vi "Dashboard Main.vi"() -> ()   [LabVIEW 2014]
uses:
  <vilib>/event_ctls.llb/eventvkey.ctl
  <vilib>/Rock Robotics/WPI/Dashboard/WPI_DashboardLogging Global.vi
  <vilib>/Utility/config.llb/Write Key (String).vi
  <vilib>/Utility/config.llb/Write Key (I32).vi
  <vilib>/Utility/config.llb/NI_LVConfig.lvlib
panel:
  in  "TCP":refnum<k5>
  in  "Rec Mode":enum32{"Stop", "Record", "Playback"}(radio)
  in  "Vision":u16(ring) items=["Camera Off", "USB Camera SW", "USB Camera HW", "IP Camera"]
  out "Camera IP":string
  out "Image Message":string="Timeout in Camera Communications"
  in  "Dashboard Tab":T1(tab)
  in  "Camera Settings":T2={"Frame Rate"=30, "Compression"=30, "Size"=1} {"Frame Rate" scale=1.0..30.0; "Size" items=["640x480", "320x240", "160x120"]}
  out "MotorChart R":cluster{"Numeric":dbl, "Numeric":dbl}(graph)
  out "MotorChart L":T3(graph)
  out "MotorSliders R":cluster{"MotorSlide1":dbl, "MotorSlide2":dbl} {"MotorSlide2" scale=-1.0..1.0 scale format="%#_2e"; "MotorSlide1" scale=-1.0..1.0 scale format="%#_2e"}
  out "MotorSliders L":T4 {"MotorSlide4 2" scale=0.0..14.0 scale format="%#_2e"; "MotorSlide2" scale=-1.0..1.0 scale format="%#_2e"; "MotorSlide1" scale=-1.0..1.0 scale format="%#_2e"}
  out "JS1 Z":dbl(slide) scale=-1.0..1.0 scale format="%#_2e"
  out "JS1 Graph":cluster{"X":dbl, "Y":dbl}[](graph)
  out "JS1 Buttons":T5
  out "JS2 Z":dbl(slide) scale=-1.0..1.0 scale format="%#_2e"
  out "JS2 Graph":cluster{"X":dbl, "Y":dbl}[](graph)
  out "JS2 Buttons":T5
  out "Mode":T6(ring)=enum."Auto Disabled"
  in  "DB Camera Config":bool
  out "fps":dbl format="%#.1g"
  out "Mbps":dbl format="%#.1g"
  out "Mbps 2":bool
  in  "DB/String 9":string
  in  "DB/String 8":string
  in  "DB/String 7":string
  in  "DB/String 6":string
  in  "DB/String 5":string
  in  "DB/String 4":string
  in  "DB/String 3":string
  in  "DB/String 2":string
  in  "DB/String 1":string
  in  "DB/String 0":string
  in  "DB/Slider 0":dbl(slide) scale=0.0..5.0
  in  "DB/Slider 1":dbl(slide) scale=0.0..5.0
  in  "DB/Slider 2":dbl(slide) scale=0.0..5.0
  in  "DB/Slider 3":dbl(slide) scale=0.0..5.0
  out "DB/LED 3":bool
  out "DB/LED 2":bool
  out "DB/LED 1":bool
  out "DB/LED 0":bool
  in  "DB/Button 3":bool
  in  "DB/Button 2":bool
  in  "DB/Button 1":bool
  in  "DB/Button 0":bool caption="New Name"
  in  "Test Slider":dbl(slide) scale=0.0..100.0 scale format="%#_3g"
  in  "On/Off":bool caption="Solenoid"
  in  "Test Name":u16(ring) items=["Select the test to run...", "Example Test", "-------------------------------", "List of tests is built in robot code.", "Replace with your own automated tests."]
  in  "Test Tree":string(tree)
  in  "Motor":cluster{"Value":dbl, "Enable":bool} {"Value" scale=-1.0..1.0 scale format="%#_3g"}
  out "Progress":T7 {"Test Progress" scale=0.0..100.0}
  in  "Rev/Fwd":cluster{"Forward":bool, "Reverse":bool}
  in  "Test Ring":u16(ring) items=["Monochrome", "Color"]
  in  "Listbox":i32(listbox)
  out "Tree":string(tree)
  out "Camera Image":T8(plugin-control)
  out "Boolean":bool
  # "Left"
  # "Front"
  # "Right"
  # "Battery"
  # "v 1.0"
  # "This tab is a great place for autonomous settings and robot-specific values.\nPlace controls and indicators inside this tab and match name to\nDashboard Variables on robot. You can also delete this comment."
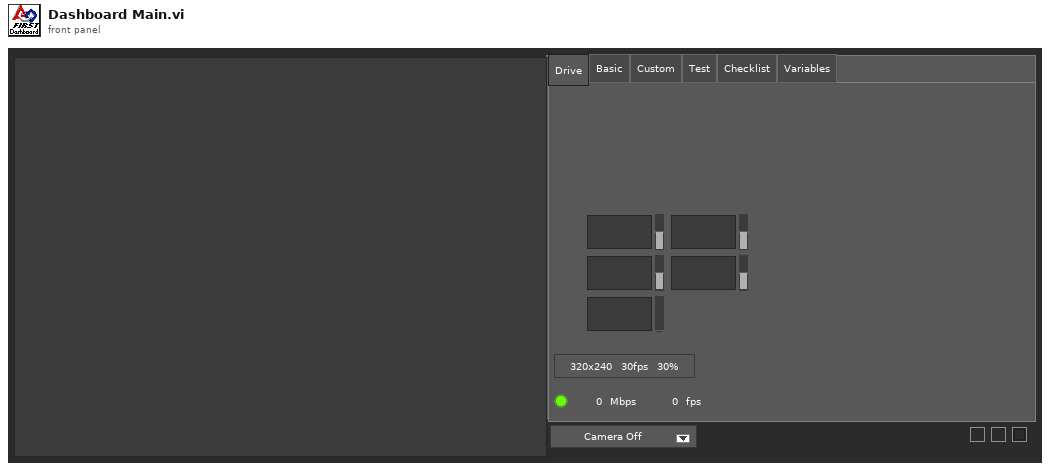
[diagram p1: front panel]
types:
  T1 = enum32{"Drive", "Basic", "Custom", "Test", "Checklist", "Variables"}
  T2 = cluster{"Frame Rate":i32, "Compression":i32, "Size":u16}
  T3 = cluster{"Numeric":dbl, "Numeric":dbl, "Battery V":dbl}
  T4 = cluster{"MotorSlide1":dbl, "MotorSlide2":dbl, "MotorSlide4 2":dbl}
  T5 = cluster{bool, bool, bool, bool, bool, bool, bool, bool, bool, bool, bool, bool}
  T6 = enum8{"Tele-Op Disabled", "Tele-Op Enabled", "Auto Disabled", "Auto Enabled", "Test Disabled", "Test Enabled", "Disconnected", "No Code", "E-Stop"}
  T7 = cluster{"Test Progress":u8, "Test Progress Text":string}
  T8 = typedef "IMAQ Image.ctl" = refnum<image>
  T9 = typedef "Image Type" = u32
  T10 = cluster{"Camera Image":refnum<vi>, "Dashboard Tab":refnum<vi>, "Boolean":refnum<vi>, "Vision":refnum<vi>, "Rec Mode":refnum<vi>, "Test Slider":refnum<vi>, "On/Off ":refnum<vi>, "Test Ring":refnum<vi>, "Rev/Fwd":refnum<vi>, "Test Name":refnum<vi>, "Motor":refnum<vi>, "Progress":refnum<vi>, "CheckList":refnum<vi>, "Tree":refnum<vi>, "Test Tree":refnum<vi>}
  T11 = cluster{"Error Strings":string, "Disable Counts":cluster{u16, u16}, "Rail Faults":cluster{u16, u16, u16}, "Robot IP":string, "DB Mode":u8, "Event Info":cluster{"Name":string, "Type":u8, "Number":u16, "Replay":u8}, "Camera Addr":string}
  T12 = cluster{"Storage":cluster{"Disk Free":u64, "RAM Block":u32, "RAM free":u32}, "CPU Utilization":cluster{"CPU % ISR":sgl, "CPU % Time Crit":sgl, "CPU % Timed Str":sgl, "CPU % High":sgl, "CPU % Above":sgl, "CPU % Normal":sgl, "CPU % Low":sgl}, "CAN":cluster{"% Bus Utilization":sgl, "Bus Off Cnt":u32, "TX_FIFO Full Cnt":u32, "Receive Error Cnt":u8, "Transmit Error Cnt":u8}, "HID":cluster{"HID Outputs":u32, "Rumble Low":u16, "Rumble High":u16}[]}
  T13 = cluster{"Status bits":cluster{"Test Mode":bool, "Autonomous":bool, "Enabled":bool, "Code Start":bool, "Brownout":bool, "Reserved 2":bool, "Reserved 3":bool, "E-Stop":bool}, "Code Trace":cluster{"Disabled":bool, "TeleOp":bool, "Auto":bool, "Test":bool}, "Controller Type":enum16{"unknown", "cRIO", "roboRio"}, "Code?":enum16{"unknown", "noCode", "code"}, "Battery V":dbl}
  T14 = cluster{"Control Bits":cluster{"TestMode":bool, "Autonomous":bool, "Enabled":bool, "FMS Present":bool, bool, bool, bool, "E-Stop":bool}, "Team Station ":u8, "Countdown":sgl, "Joystick Values":cluster{"Axes":dbl[], "Buttons":bool[], "POVs":i16[]}[]}
  T15 = cluster{"Axes":dbl[], "Buttons":bool[], "POVs":i16[]}[]
  T16 = cluster{"Axes":dbl[], "Buttons":bool[], "POVs":i16[]}
  T17 = cluster{"Buttons[0]":bool, "Buttons[1]":bool, "Buttons[2]":bool, "Buttons[3]":bool, "Buttons[4]":bool, "Buttons[5]":bool, "Buttons[6]":bool, "Buttons[7]":bool, "Buttons[8]":bool, "Buttons[9]":bool, "Buttons[10]":bool, "Buttons[11]":bool}
  T18 = typedef "NI_LVConfig.lvlib/Config Data RefNum.ctl" = refnum<k1>
  T19 = cluster{"Operation":enum16{"Update", "Clear"}, "Color Box":u32}[]
  T20 = typedef "eventvkey.ctl" = enum16{"ASCII", "Enter", "Return", "Shift", "Ctrl", "Alt", "Cmd", "Opt", "Caps", "NumLock", "Clear", "Break", "Up", "Down", "Left", "Right", "Insert", "Delete", "Home", "End", "PageUp", "PageDown", "Escape", "Help", "Pause", "ScrollLock", "F1", "F2", "F3", "F4", "F5", "F6", "F7", "F8", "F9", "F10", "F11", "F12", "F13", "F14", "F15", "F16", "F17", "F18", "F19", "F20", "F21", "F22", "F23", "F24", "Play", "VolumeUp", "VolumeDown", "Mute", "Two Byte Char"}
  T21 = cluster{"Image Size":bool, "Image Type":bool, "Pixel Value":bool, "ROI Information":bool, "Zoom Factor":bool}
  T22 = enum8{"Enabled", "Disabled", "Disabled and Grayed Out"}
  T23 = cluster{"Operation":enum16{"Update", "Clear"}, "Color Box":u32}
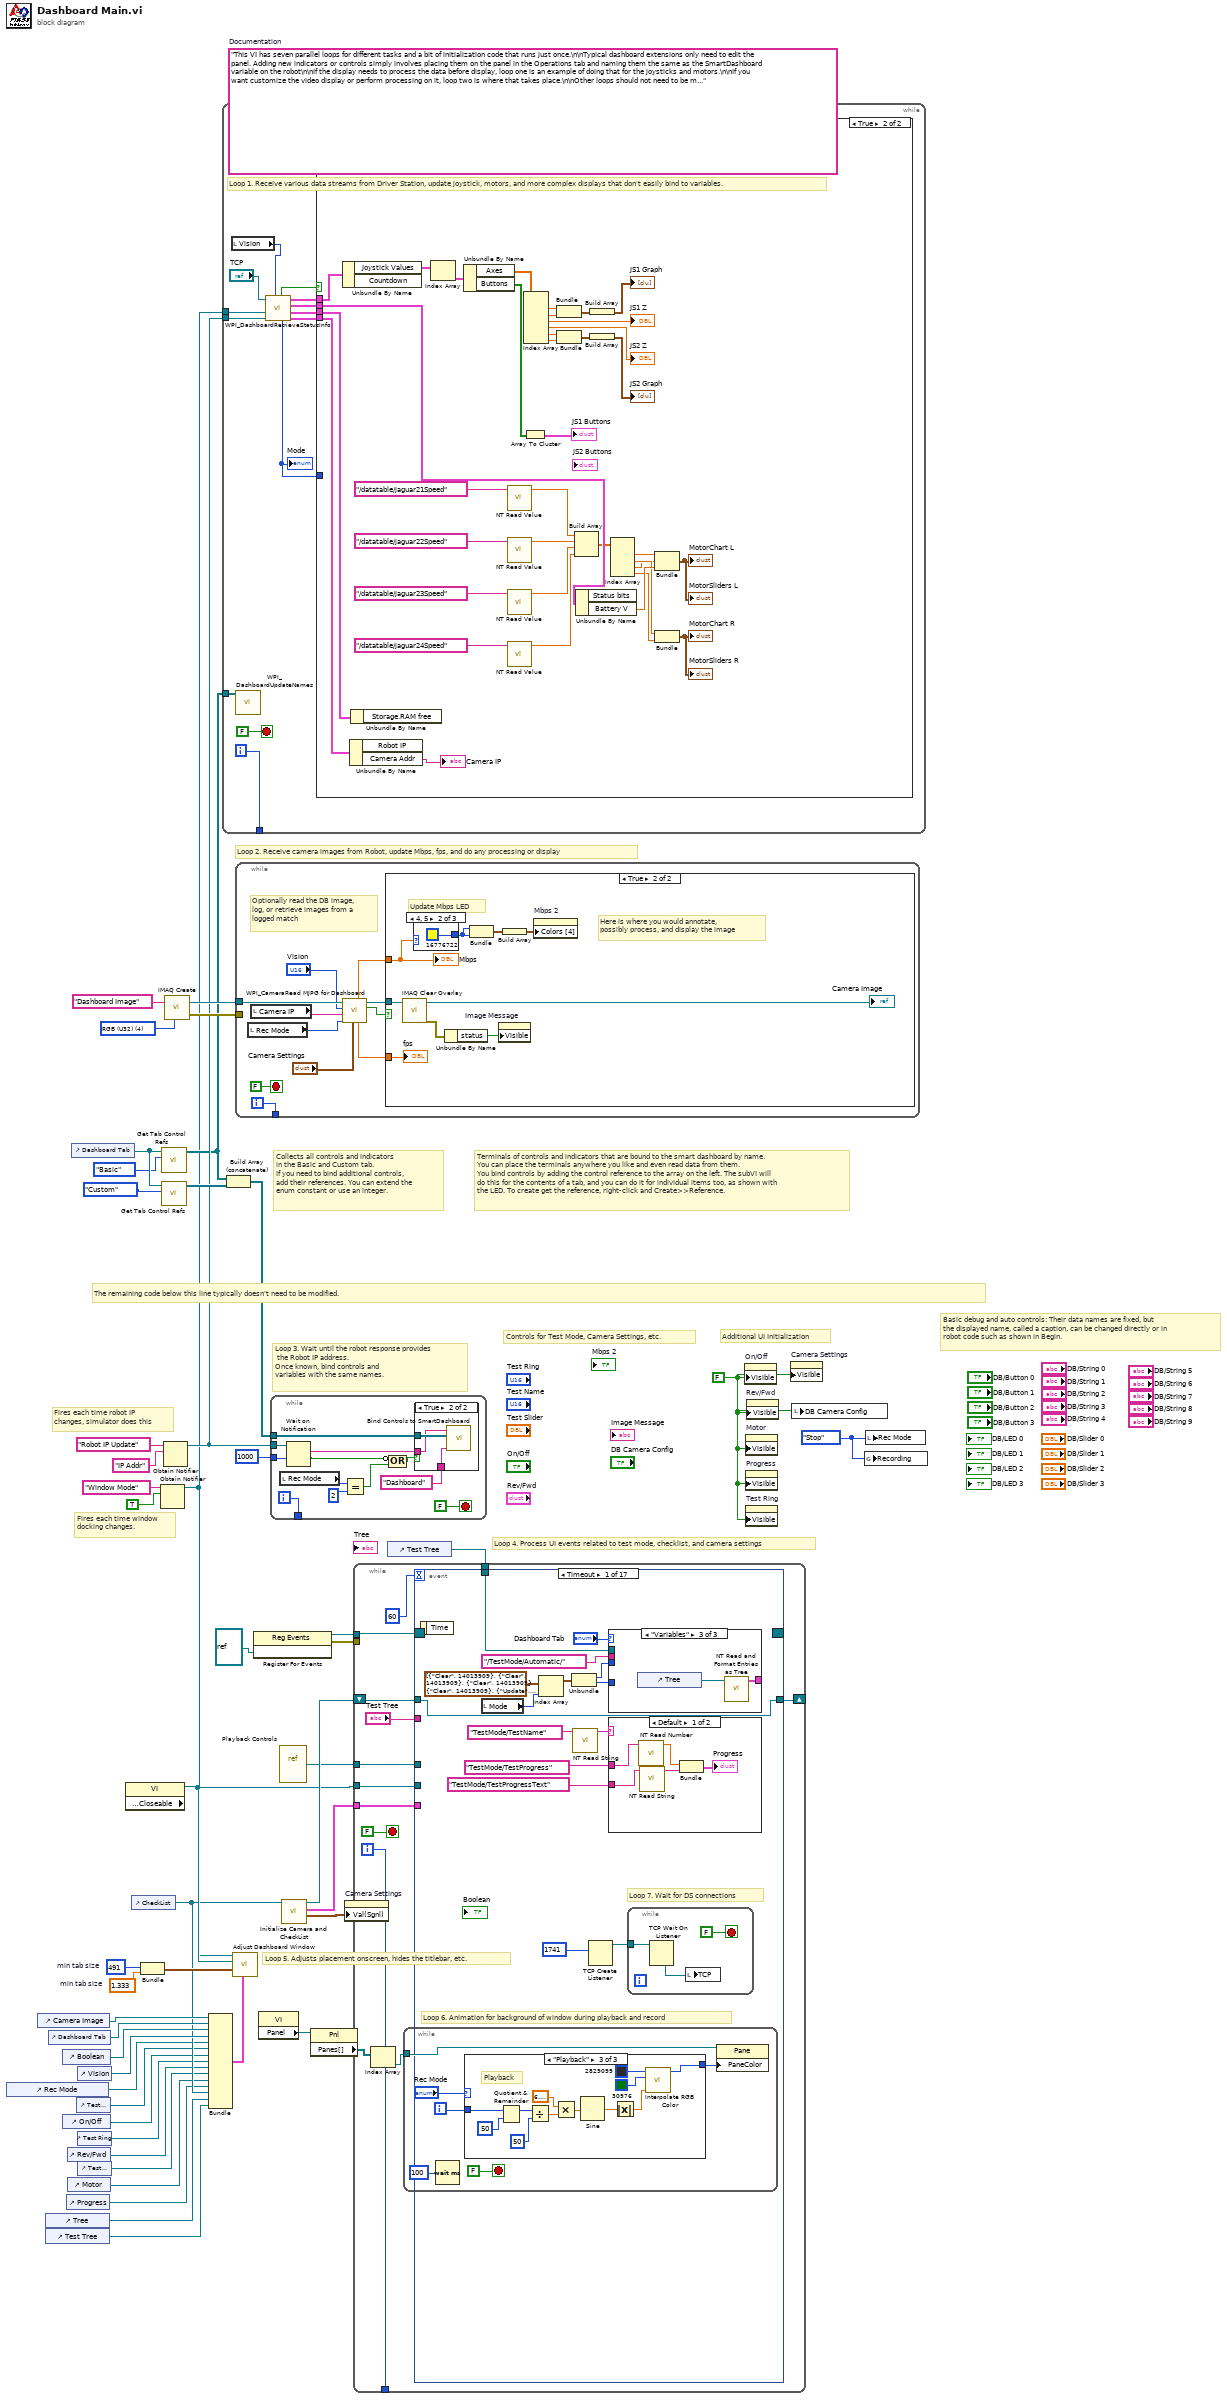
[diagram p0: block diagram]
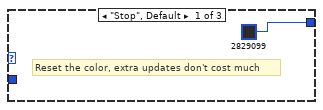
[diagram p3: hidden frame]
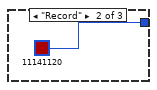
[diagram p4: hidden frame]
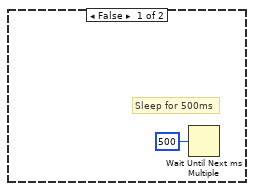
[diagram p6: hidden frame]
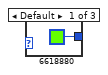
[diagram p7: hidden frame]
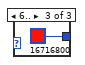
[diagram p8: hidden frame]
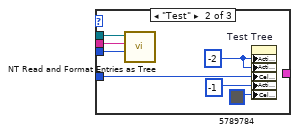
[diagram p10: hidden frame]
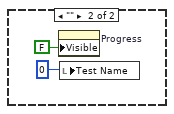
[diagram p11: hidden frame]
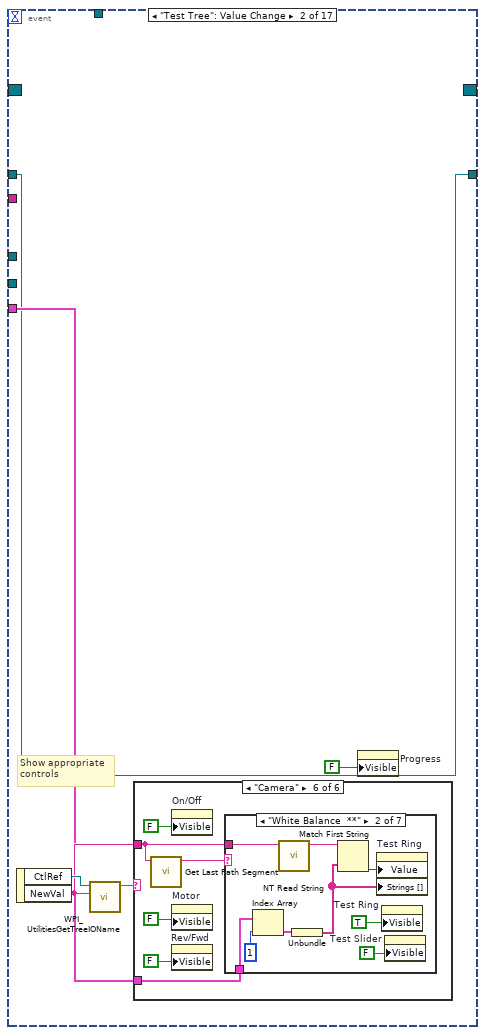
[diagram p12: hidden frame]
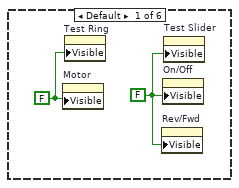
[diagram p13: hidden frame]
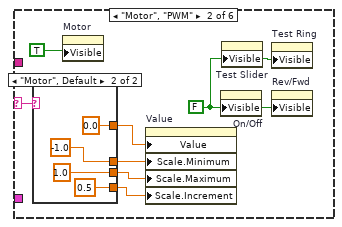
[diagram p14: hidden frame]
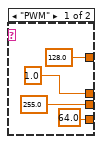
[diagram p15: hidden frame]
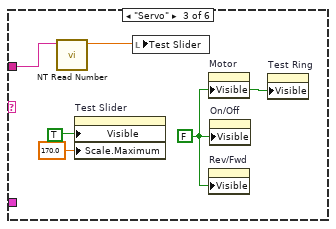
[diagram p16: hidden frame]
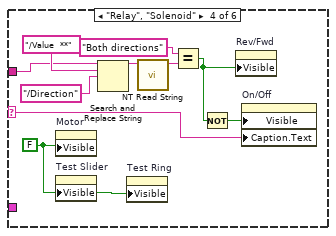
[diagram p17: hidden frame]
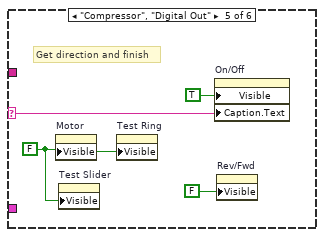
[diagram p18: hidden frame]
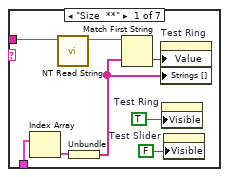
[diagram p19: hidden frame]
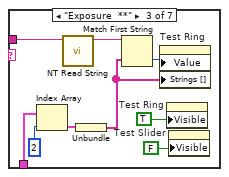
[diagram p20: hidden frame]
diagram:
  w24 = 491  # min tab size
  w23 = 1.333  # min tab size
  w32 = enum32{"Stop", "Record", "Playback"}."Stop" ("Rec Mode")
  w6 = FALSE ("Visible")
  (unwired) "This VI has seven parallel loops for different tasks and a bit of initialization code that runs just once.\n\nTypical dashboard extensions only need to edit the panel. Adding new indicators or controls simply involves placing them on the panel in the Operations tab and naming them the same as the SmartDashboard variable on the robot\n\nIf the display needs to process the data before display, loop one is an example of doing that for the joysticks and motors.\n\nIf you want customize the video display or perform processing on it, loop two is where that takes place.\n\nOther loops should not need to be modified. They are pretty standard, and document the task they perform."  # Documentation
  w52 = T9 4 items=["Grayscale (U8)", "Grayscale (I16)", "Grayscale (SGL)", "Complex (CSG)", "RGB (U32)", "HSL (U32)", "RGB (U64)"] ("Image Type")
  # "Loop 7. Wait for DS connections"
  # "Basic debug and auto controls: Their data names are fixed, but\nthe displayed name, called a caption, can be changed directly or in\nrobot code such as shown in Begin."
  # "Controls for Test Mode, Camera Settings, etc."
  # "Additional UI Initialization"
  # "Loop 6. Animation for background of window during playback and record"
  # "Fires each time robot IP\nchanges, simulator does this"
  # "Fires each time window\ndocking changes."
  # "Collects all controls and indicators\nin the Basic and Custom tab.\nIf you need to bind additional controls,\nadd their references. You can extend the\nenum constant or use an integer."
  # "The remaining code below this line typically doesn't need to be modified."
  # "Loop 4. Process UI events related to test mode, checklist, and camera settings"
  # "Terminals of controls and indicators that are bound to the smart dashboard by name.\nYou can place the terminals anywhere you like and even read data from them.\nYou bind controls by adding the control reference to the array on the left. The subVI will\ndo this for the contents of a tab, and you can do it for individual items too, as shown with\nthe LED. To create get the reference, right-click and Create>>Reference."
  # "Loop 3. Wait until the robot response provides\n the Robot IP address.\nOnce known, bind controls and\nvariables with the same names."
  # "Loop 5. Adjusts placement onscreen, hides the titlebar, etc."
  # "Loop 1. Receive various data streams from Driver Station, update joystick, motors, and more complex displays that don't easily bind to variables."
  # "Loop 2. Receive camera images from Robot, update Mbps, fps, and do any processing or display"
  n1 = control-ref of="Rec Mode"() -> (w12:refnum<vi>)
  n2 = control-ref of="Camera Image"() -> (w27:refnum<vi>)
  n3 = control-ref of="Tree"() -> (w16:refnum<vi>)
  n4 = control-ref of="Test Tree"() -> (w15:refnum<vi>)
  n5 = control-ref of="Dashboard Tab"() -> (w26:refnum<vi>)
  n6 = control-ref of="Boolean"() -> (w21:refnum<vi>)
  n7 = control-ref of="On/Off"() -> (w10:refnum<vi>)
  n8 = control-ref of="Progress"() -> (w7:refnum<vi>)
  n9 = control-ref of="Rev/Fwd"() -> (w8:refnum<vi>)
  n10 = control-ref of="Motor"() -> (w13:refnum<vi>)
  n11 = control-ref of="Dashboard Tab"() -> (w30:refnum<vi>)
  n12 = control-ref of="Test Slider"() -> (w11:refnum<vi>)
  n13 = control-ref of="Vision"() -> (w25:refnum<vi>)
  n14 = control-ref of="Test Ring"() -> (w9:refnum<vi>)
  n15 = control-ref of="Test Name"() -> (w14:refnum<vi>)
  n16 = property class="VI" props=["Front Panel.Closeable"]() -> (reference out=w31:refnum<vi>)  [unwired: 2 in, 2 out]
  n17 = control-ref of="CheckList"() -> (w17:refnum<vi>)
  n18 = Bundle("min tab size"=w24, "min tab size"=w23) -> (w22:cluster{"min tab size":i32, "min tab size":dbl})  [unwired: 1 in]
  n19 = Obtain Notifier(name (unnamed)="Window Mode", notification data type=TRUE) -> (notifier out=w3:refnum<notifier>)  [unwired: 2 in, 2 out]
  n20 = call <vilib>:"Get Tab Control Refs.vi"("Page Index"=T1."Basic" ("Dashboard Tab"), "TabControl in"=w30) -> ("ControlsOnPage"=w4:refnum<vi>[])  [unwired: 9 in]
  n21 = call <vilib>:"Get Tab Control Refs.vi"("Page Index"=T1."Custom" ("Dashboard Tab"), "TabControl in"=w30) -> ("ControlsOnPage"=w29:refnum<vi>[])  [unwired: 9 in]
  n22 = Obtain Notifier(name (unnamed)="Robot IP Update", notification data type="IP Addr" ("name (unnamed)")) -> (notifier out=w5:refnum<notifier>)  [unwired: 2 in, 2 out]
  n23 = call "IMAQ Create"("Image Name"="Dashboard Image", "Image Type"=w52) -> ("New Image"=w50:T8, "error out"=w49:errorcluster)  [unwired: 2 in, 1 out]
  n24 = Bundle("Camera Image"=w27, "Dashboard Tab"=w26, "Boolean"=w21, "Vision"=w25, "Rec Mode"=w12, "Test Slider"=w11, "On/Off"=w10, "Test Ring"=w9, "Rev/Fwd"=w8, "Test Name"=w14, "Motor"=w13, "Progress"=w7, "CheckList"=w17, "Tree"=w16, "Test Tree"=w15) -> (w18:T10)  [unwired: 1 in]
  n25 = while {
    tunnel: [w64] -> _
    tunnel: w5 -> [w58]
    tunnel: w4 -> [w57]
    tunnel: w3 -> [w53]
    i -> [w64]
    stop <- FALSE stop-if-true
    n26 = local read "Vision"() -> (w55:u16)
    n27 = call <vilib>:"WPI_DashboardUpdateNames.vi"("Controls on Tab"=w57) -> ()  [unwired: 11 in]
    n28 = call <vilib>:"WPI_DashboardRetrieveStatusInfo.vi"("Vision"=w55, "Binding Refnum"=w58, "Window Mode Notifier"=w53, "TCP Cnx"="TCP") -> ("Power and Errors"=w59:T11, "Robot Metrics"=w62:T12, "Status Info"=w63:T13, "Control Info"=w60:T14, "Robot Mode"=w56:T6, "Process?"=w61:bool)  [unwired: 2 in]
    "Mode" <- w56
    n29 = case shown="True" w61 {
      tunnel: w63 -> [_ w101]
      tunnel: w62 -> [_ w100]
      tunnel: w60 -> [_ w99]
      tunnel: w59 -> [_ w98]
      tunnel: w56 -> [_ _]
      frame False {
      }
      frame True {
        n30 = Unbundle By Name(w99) -> ("Joystick Values"=w94:T15)  [unwired: 1 out]
        n31 = Unbundle By Name(w98) -> ("Camera Addr"=→"Camera IP":string)  [unwired: 1 out]
        n32 = Unbundle By Name(w100) -> ()  [unwired: 1 out]
        n33 = Index Array(array=w94) -> (element=w92:T16)  [unwired: 1 in]
        n34 = Unbundle By Name(w92) -> ("Axes"=w88:dbl[], "Buttons"=w87:bool[])
        n35 = call-poly <vilib>:"NT Read Value.vi"("Name"="/datatable/jaguar21Speed") -> ("Numeric"=w74:dbl)  [unwired: 9 in, 1 out]
        n36 = call-poly <vilib>:"NT Read Value.vi"("Name"="/datatable/jaguar22Speed") -> ("Numeric"=w73:dbl)  [unwired: 9 in, 1 out]
        n37 = call-poly <vilib>:"NT Read Value.vi"("Name"="/datatable/jaguar23Speed") -> ("Numeric"=w71:dbl)  [unwired: 9 in, 1 out]
        n38 = call-poly <vilib>:"NT Read Value.vi"("Name"="/datatable/jaguar24Speed") -> ("Numeric"=w70:dbl)  [unwired: 9 in, 1 out]
        n39 = Array To Cluster(array=w87) -> (cluster=→"JS1 Buttons":T17)
        n40 = Index Array(array=w88) -> (element #1=w90:dbl, element #2=w91:dbl, element #3=→"JS1 Z":dbl, element #4=→"JS2 Z":dbl, element #5=w67:dbl, element #6=w66:dbl)  [unwired: 6 in]
        n41 = Bundle("X axis"=w90, "X axis"=w91) -> (w89:cluster{"X axis":dbl, "X axis":dbl})  [unwired: 1 in]
        n42 = Bundle("X axis"=w67, "X axis"=w66) -> (w84:cluster{"X axis":dbl, "X axis":dbl})  [unwired: 1 in]
        n43 = Build Array(w74, w73, w71, w70) -> (w72:dbl[])
        n44 = Unbundle By Name(w101) -> ("Battery V"=w95:dbl)  [unwired: 1 out]
        n45 = Build Array(w89) -> (→"JS1 Graph":cluster{"X axis":dbl, "X axis":dbl}[])
        n46 = Build Array(w84) -> (→"JS2 Graph":cluster{"X axis":dbl, "X axis":dbl}[])
        n47 = Index Array(array=w72) -> (element #1=w82:dbl, element #2=w81:dbl, element #3=w80:dbl, element #4=w79:dbl)  [unwired: 4 in]
        n48 = Bundle("Numeric"=w82, "Numeric"=w80, "Battery V"=w95) -> (→"MotorChart L" →"MotorSliders L":T3)  [unwired: 1 in]
        n49 = Bundle("Numeric"=w81, "Numeric"=w79) -> (→"MotorChart R" →"MotorSliders R":cluster{"Numeric":dbl, "Numeric":dbl})  [unwired: 1 in]
      }
    }
  }
  n50 = Build Array (concatenate)(w4, w29) -> (w28:refnum<vi>[])
  n51 = call "Adjust Dashboard Window.vi"("Sizing Refnums"=w18, "Size Constraints"=w22, "VI"=w31, "Notifier in"=w3) -> ()  [unwired: 8 in]
  n52 = while {
    tunnel: w50 -> [w110]
    tunnel: w49 -> [_]
    tunnel: [w111] -> _
    i -> [w111]
    stop <- FALSE stop-if-true
    # "Optionally read the DB image,\nlog, or retrieve images from a\nlogged match"
    n53 = local read "Rec Mode"() -> (w104:enum32{"Stop", "Record", "Playback"})
    n54 = local read "Camera IP"() -> (w102:string)
    n55 = call <vilib>:"WPI_CameraRead MJPG for Dashboard.vi"("Camera Settings"="Camera Settings", "Rec Mode"=w104, "Camera IP"=w102, "Camera Mode"="Vision", "Refnum in"=w110) -> ("Active"=w108:bool, "Refnum out"=w109:T8, "FPS"=w107:dbl, "Bandwidth (Mbps)"=w106:dbl)  [unwired: 3 in]
    n56 = case shown="True" w108 {
      tunnel: w109 -> [_ w117]
      tunnel: w106 -> [_ w116]
      tunnel: w107 -> [_ w114]
      frame False {
        # "Sleep for 500ms"
        n57 = Wait Until Next ms Multiple(millisecond multiple=u32 500) -> ()  [unwired: 1 out]
      }
      frame True {
        # "Here is where you would annotate,\npossibly process, and display the image"
        # "Update Mbps LED"
        n58 = call "IMAQ Clear Overlay"("Image"=w117) -> ("error out"=w121:errorcluster, "Image Out"=→"Camera Image":T8)  [unwired: 2 in, 7 out]
        n59 = case shown="4, 5" w116 {
          tunnel: [u32 6618880 ("Color Box") u32 16776722 ("Color Box") u32 16716800 ("Color Box")] -> w118
          frame Default {
          }
          frame 4, 5 {
          }
          frame 6.. {
          }
        }
        n60 = Unbundle By Name(w121) -> ("status"=w122:bool)
        n61 = Bundle("Color Box"=w118, "Color Box"=w118) -> (w120:cluster{"Color Box":u32, "Color Box":u32})  [unwired: 1 out]
        n62 = property on="Image Message" class="Str"("Visible"=w122) -> ()  [unwired: 2 in, 2 out]
        n63 = Build Array(w120) -> (w119:cluster{"Color Box":u32, "Color Box":u32}[])
        n64 = property on="Mbps 2" class="Bool (strict)"("Colors [4]"=w119) -> ()  [unwired: 2 in, 2 out]
        "Mbps" <- w116
        "fps" <- w114
      }
    }
  }
  n65 = register-events(refnum<vi> refnum) -> (reference out=w36:refnum<event-registration>, error out=w35:errorcluster)  [unwired: 2 in]
  n66 = property class="VI"() -> ("Panel"=w39:refnum<vi>)  [unwired: 2 in, 2 out]
  n67 = while {
    tunnel: w28 -> [w137]
    tunnel: w5 -> [w135]
    tunnel: [w133] -> _
    tunnel: u32 1000 ("milliseconds to wait") -> [w132]
    i -> [w133]
    stop <- FALSE stop-if-true
    n68 = local read "Rec Mode"() -> (w128:enum32{"Stop", "Record", "Playback"})
    n69 = Wait on Notification(notifier=w135, timeout in ms (-1)=w132) -> (notification=w134:string, timed out?=w130:bool)  [unwired: 2 in, 2 out]
    n70 = Equal?(x=w128, y=u16 2 ("Rec Mode")) -> (x = y?=w129:bool)
    n71 = Compound Arithmetic op=OR(invert w130, w129) -> (w131:bool)
    n72 = case shown="True" w131 {
      tunnel: w137 -> [_ w140]
      tunnel: w134 -> [_ w139]
      tunnel: "Dashboard" -> [_ w138]
      frame False {
      }
      frame True {
        n73 = call <vilib>:"Bind Controls to SmartDashboard.vi"("Client Name"=w138, "Bound Control Refs"=w140, "Server IP Address"=w139) -> ()  [unwired: 9 in]
      }
    }
  }
  n74 = vi-ref "Playback Controls.vi"() -> (w37:refnum<vi>)
  n75 = call "Initialize Camera and CheckList.vi"("ListBox in"=w17) -> ("Cluster"=w43:cluster{"value":i32, "value":i32, "index":i32}, "Array"=w44:cluster{string[]}[], "File Refnum"=w42:T18)  [unwired: 8 in]
  n76 = property class="Pnl"(reference=w39) -> ("Panes[]"=w40:refnum<vi>[])  [unwired: 1 in, 2 out]
  n77 = property on="Camera Settings" class="Clust (strict)"("Val(Sgnl)"=w43) -> ()  [unwired: 2 in, 2 out]
  n78 = Index Array(array=w40) -> (element=w38:refnum<vi>)  [unwired: 1 in]
  n79 = control-ref of="Test Tree"() -> (w41:refnum<vi>)
  n80 = while {
    tunnel: w44 -> [w148]
    shift-right: [w147] -> _
    shift-left: w42 -> [w146]
    tunnel: [w145] -> _
    tunnel: w41 -> [w144]
    tunnel: w37 -> [w143]
    tunnel: w36 -> [w142]
    tunnel: w35 -> [_]
    tunnel: w31 -> [w141]
    i -> [w145]
    stop <- FALSE stop-if-true
    n81 = event shown="[0] Timeout" {
      selector: w142 -> [_ _ _ _ _ _ _ _ _ _ _ _ _ _ _ _ _]
      dyn-events: [_ _ _ _ _ _ _ _ _ _ _ _ _ w386 _ _ _] -> _
      timeout: u32 60 ("milliseconds to wait") -> [_ _ _ _ _ _ _ _ _ _ _ _ _ _ _ _ _]
      tunnel: w144 -> [w160 _ _ _ _ _ _ _ _ _ _ _ _ _ _ _ _]
      tunnel: "Test Tree" -> [_ _ _ _ _ _ _ _ w355 w363 w365 w369 w377 _ _ _ _]
      tunnel: w148 -> [_ w182 _ _ _ _ w319 w349 _ _ _ _ _ _ _ _ _]
      tunnel: [w156 w181 w280 w285 w293 w305 w318 w342 w354 w361 w364 w368 w376 w388 w402 w403 w413] -> w147
      tunnel: w146 -> [w156 w181 w280 w285 w293 w305 w317 w342 w354 w361 w364 w368 w376 w388 w402 w403 w413]
      tunnel: w143 -> [_ _ _ _ _ _ _ _ _ _ _ _ _ w389 _ w406 _]
      tunnel: w141 -> [_ _ _ _ _ _ _ _ _ _ _ _ _ w384 _ _ _]
      event Timeout {
        n82 = event-data() -> ()  [unwired: 1 in, 1 out]
        n83 = local read "Mode"() -> (w159:T6)
        n84 = Index Array(array=T19 [{"Operation"=enum."Clear", "Color Box"=14013909}, {"Operation"=enum."Clear", "Color Box"=14013909}, {"Operation"=enum."Clear", "Color Box"=14013909}, {"Operation"=enum."Clear", "Color Box"=14013909}, {"Operation"=enum."Update", "Color Box"=14013909}, {"Operation"=enum."Update", "Color Box"=16777215}, {"Operation"=enum."Clear", "Color Box"=14013909}, {"Operation"=enum."Clear", "Color Box"=14013909}, {"Operation"=enum."Clear", "Color Box"=14013909}], index=w159) -> (element=w154:T23)
        n85 = Unbundle(w154) -> ("Operation"=w153:enum16{"Update", "Clear"}, "Color Box"=w152:u32)
        n86 = call <vilib>:"NT Read String.vi"("Name"="TestMode/TestName") -> ("String"=w163:string)  [unwired: 9 in, 1 out]
        n87 = case shown="\"Variables\"" "Dashboard Tab" {
          tunnel: w160 -> [_ w171 _]
          tunnel: "/TestMode/Automatic/" ("Name Pattern") -> [_ w170 _]
          tunnel: w153 -> [_ w169 _]
          tunnel: [_ _ w173] -> _
          tunnel: w152 -> [_ w165 _]
          frame "Custom", Default {
          }
          frame "Test" {
            w168 = -2 ("Active Item:Row Number")
            n88 = call <vilib>:"NT Read and Format Entries as Tree.vi"("Operation"=w169, "Name Pattern"=w170, "Tree Refnum"=w171) -> ()  [unwired: 7 in, 2 out]
            n89 = property on="Test Tree" class="Tree (strict)"("Active Item Row Number"=w168, "ActiveColNum"=w168, "CellBG"=w165, "Active Item Row Number"=-1 ("Active Item:Row Number"), "CellBG"=u32 5789784 ("Color Box")) -> ()  [unwired: 2 in, 2 out]
          }
          frame "Variables" {
            n90 = control-ref of="Tree"() -> (w172:refnum<vi>)
            n91 = call <vilib>:"NT Read and Format Entries as Tree.vi"("Tree Refnum"=w172) -> ("Formatted Strings"=w173:cluster{"Name":string, "Value":string}[])  [unwired: 9 in, 1 out]
          }
        }
        n92 = case shown="Default" w163 {
          tunnel: "TestMode/TestProgress" ("Name") -> [w175 _]
          tunnel: "TestMode/TestProgressText" ("Name") -> [w174 _]
          frame Default {
            n93 = call <vilib>:"NT Read Number.vi"("Name"=w175) -> ("Numeric"=w176:dbl)  [unwired: 9 in, 1 out]
            n94 = call <vilib>:"NT Read String.vi"("Name"=w174) -> ("String"=w177:string)  [unwired: 9 in, 1 out]
            n95 = Bundle("Numeric"=w176, "String"=w177) -> (→"Progress":cluster{"Numeric":dbl, "String":string})  [unwired: 1 in]
          }
          frame "" {
            n96 = property on="Progress" class="Clust (strict)"("Visible"=FALSE) -> ()  [unwired: 2 in, 2 out]
            n97 = local write "Test Name"(u16 0) -> ()
          }
        }
      }
      event "Test Tree": Value Change {
        # "Show appropriate\ncontrols"
        n98 = event-data() -> ("CtlRef"=w185:refnum<vi>, "NewVal"=w183:string)  [unwired: 1 in]
        n99 = call <vilib>:"WPI_UtilitiesGetTreeIOName.vi"("NewVal"=w183, "TreeControl in"=w185) -> ("I/O Name"=w186:string)  [unwired: 9 in]
        n100 = case shown="\"Camera\"" w186 {
          selector: w186 -> [_ w193 _ w211 w220 _]
          tunnel: w183 -> [_ _ w208 w210 _ w227]
          tunnel: w182 -> [_ _ _ _ _ w226]
          frame Default {
            w188 = FALSE ("Visible")
            w187 = FALSE ("Visible")
            n101 = property on="Motor" class="Clust (strict)"("Visible"=w187) -> ()  [unwired: 2 in, 2 out]
            n102 = property on="Test Ring" class="Ring (strict)"("Visible"=w187) -> ()  [unwired: 2 in, 2 out]
            n103 = property on="Rev/Fwd" class="Clust (strict)"("Visible"=w188) -> ()  [unwired: 2 in, 2 out]
            n104 = property on="On/Off" class="Bool (strict)"("Visible"=w188) -> ()  [unwired: 2 in, 2 out]
            n105 = property on="Test Slider" class="Slide (strict)"("Visible"=w188) -> ()  [unwired: 2 in, 2 out]
          }
          frame "Motor", "PWM" {
            w194 = FALSE ("Visible")
            n106 = case shown="\"Motor\", Default" w193 {
              tunnel: [1.0 ("Value") -1.0 ("Value")] -> w192
              tunnel: [255.0 ("Value") 1.0 ("Value")] -> w191
              tunnel: [128.0 ("Value") 0.0 ("Value")] -> w190
              tunnel: [64.0 ("Value") 0.5 ("Value")] -> w189
              frame "PWM" {
              }
              frame "Motor", Default {
              }
            }
            n107 = property on="Motor" class="Clust (strict)"("Visible"=TRUE) -> ()  [unwired: 2 in, 2 out]
            n108 = property on="Value" class="Slide (strict)"("Value"=w190, "Scale.Minimum"=w192, "Scale.Maximum"=w191, "Scale.Increment"=w189) -> ()  [unwired: 2 in, 2 out]
            n109 = property on="On/Off" class="Bool (strict)"("Visible"=w194) -> ()  [unwired: 2 in, 2 out]
            n110 = property on="Test Slider" class="Slide (strict)"("Visible"=w194) -> ()  [unwired: 2 in, 2 out]
            n111 = property on="Test Ring" class="Ring (strict)"("Visible"=w194) -> ()  [unwired: 2 in, 2 out]
            n112 = property on="Rev/Fwd" class="Clust (strict)"("Visible"=w194) -> ()  [unwired: 2 in, 2 out]
          }
          frame "Servo" {
            w206 = FALSE ("Visible")
            n113 = call <vilib>:"NT Read Number.vi"("Name"=w208) -> ("Numeric"=w207:dbl)  [unwired: 9 in, 1 out]
            n114 = property on="Test Slider" class="Slide (strict)"("Visible"=TRUE, "Scale.Maximum"=170.0 ("Scale.Range:Maximum")) -> ()  [unwired: 2 in, 2 out]
            n115 = local write "Test Slider"(w207) -> ()
            n116 = property on="Motor" class="Clust (strict)"("Visible"=w206) -> ()  [unwired: 2 in, 2 out]
            n117 = property on="Rev/Fwd" class="Clust (strict)"("Visible"=w206) -> ()  [unwired: 2 in, 2 out]
            n118 = property on="On/Off" class="Bool (strict)"("Visible"=w206) -> ()  [unwired: 2 in, 2 out]
            n119 = property on="Test Ring" class="Ring (strict)"("Visible"=w206) -> ()  [unwired: 2 in, 2 out]
          }
          frame "Relay", "Solenoid" {
            w209 = FALSE ("Visible")
            n120 = property on="Motor" class="Clust (strict)"("Visible"=w209) -> ()  [unwired: 2 in, 2 out]
            n121 = property on="Test Slider" class="Slide (strict)"("Visible"=w209) -> ()  [unwired: 2 in, 2 out]
            n122 = Search and Replace String(input string=w210, search string="/Value  **", replace string="/Direction") -> (result string=w216:string)  [unwired: 5 in, 3 out]
            n123 = property on="Test Ring" class="Ring (strict)"("Visible"=w209) -> ()  [unwired: 2 in, 2 out]
            n124 = call <vilib>:"NT Read String.vi"("Name"=w216) -> ("String"=w214:string)  [unwired: 9 in, 1 out]
            n125 = Equal?(x="Both directions", y=w214) -> (x = y?=w212:bool)
            n126 = Not(x=w212) -> (.not. x?=w213:bool)
            n127 = property on="Rev/Fwd" class="Clust (strict)"("Visible"=w212) -> ()  [unwired: 2 in, 2 out]
            n128 = property on="On/Off" class="Bool (strict)"("Visible"=w213, "Caption.Text"=w211) -> ()  [unwired: 2 in, 2 out]
          }
          frame "Compressor", "Digital Out" {
            w219 = FALSE ("Visible")
            # "Get direction and finish"
            n129 = property on="Motor" class="Clust (strict)"("Visible"=w219) -> ()  [unwired: 2 in, 2 out]
            n130 = property on="Test Slider" class="Slide (strict)"("Visible"=w219) -> ()  [unwired: 2 in, 2 out]
            n131 = property on="Test Ring" class="Ring (strict)"("Visible"=w219) -> ()  [unwired: 2 in, 2 out]
            n132 = property on="On/Off" class="Bool (strict)"("Visible"=TRUE, "Caption.Text"=w220) -> ()  [unwired: 2 in, 2 out]
            n133 = property on="Rev/Fwd" class="Clust (strict)"("Visible"=FALSE) -> ()  [unwired: 2 in, 2 out]
          }
          frame "Camera" {
            n134 = call <vilib>:"Get Last Path Segment.vi"("String in"=w227) -> ("String out"=w228:string)  [unwired: 10 in]
            n135 = property on="On/Off" class="Bool (strict)"("Visible"=FALSE) -> ()  [unwired: 2 in, 2 out]
            n136 = property on="Motor" class="Clust (strict)"("Visible"=FALSE) -> ()  [unwired: 2 in, 2 out]
            n137 = property on="Rev/Fwd" class="Clust (strict)"("Visible"=FALSE) -> ()  [unwired: 2 in, 2 out]
            n138 = case shown="\"White Balance  **\"" w228 {
              tunnel: w227 -> [w234 w243 w252 w261 w270 _ w276]
              tunnel: w226 -> [w232 w240 w249 w258 w267 _ _]
              frame "Size  **" {
                n139 = Index Array(array=w232) -> (element=w231:cluster{string[]})  [unwired: 1 in]
                n140 = call <vilib>:"NT Read String.vi"("Name"=w234) -> ("String"=w233:string)  [unwired: 9 in, 1 out]
                n141 = Unbundle(w231) -> (w229:string[])
                n142 = Match First String(2:w229, 3:w233) -> (0:w230:i32)  [unwired: 1 out]
                n143 = property on="Test Ring" class="Ring (strict)"("Value"=w230, "Strings []"=w229) -> ()  [unwired: 2 in, 2 out]
                n144 = property on="Test Ring" class="Ring (strict)"("Visible"=TRUE) -> ()  [unwired: 2 in, 2 out]
                n145 = property on="Test Slider" class="Slide (strict)"("Visible"=FALSE) -> ()  [unwired: 2 in, 2 out]
              }
              frame "White Balance  **" {
                n146 = Index Array(array=w240, index=1) -> (element=w241:cluster{string[]})
                n147 = call <vilib>:"NT Read String.vi"("Name"=w243) -> ("String"=w242:string)  [unwired: 9 in, 1 out]
                n148 = Unbundle(w241) -> (w238:string[])
                n149 = Match First String(2:w238, 3:w242) -> (0:w237:i32)  [unwired: 1 out]
                n150 = property on="Test Ring" class="Ring (strict)"("Value"=w237, "Strings []"=w238) -> ()  [unwired: 2 in, 2 out]
                n151 = property on="Test Ring" class="Ring (strict)"("Visible"=TRUE) -> ()  [unwired: 2 in, 2 out]
                n152 = property on="Test Slider" class="Slide (strict)"("Visible"=FALSE) -> ()  [unwired: 2 in, 2 out]
              }
              frame "Exposure  **" {
                n153 = Index Array(array=w249, index=2) -> (element=w250:cluster{string[]})
                n154 = call <vilib>:"NT Read String.vi"("Name"=w252) -> ("String"=w251:string)  [unwired: 9 in, 1 out]
                n155 = Unbundle(w250) -> (w246:string[])
                n156 = Match First String(2:w246, 3:w251) -> (0:w247:i32)  [unwired: 1 out]
                n157 = property on="Test Ring" class="Ring (strict)"("Value"=w247, "Strings []"=w246) -> ()  [unwired: 2 in, 2 out]
                n158 = property on="Test Ring" class="Ring (strict)"("Visible"=TRUE) -> ()  [unwired: 2 in, 2 out]
                n159 = property on="Test Slider" class="Slide (strict)"("Visible"=FALSE) -> ()  [unwired: 2 in, 2 out]
              }
              frame "Exposure Priority  **" {
                n160 = Index Array(array=w258, index=3) -> (element=w259:cluster{string[]})
                n161 = call <vilib>:"NT Read String.vi"("Name"=w261) -> ("String"=w260:string)  [unwired: 9 in, 1 out]
                n162 = Unbundle(w259) -> (w255:string[])
                n163 = Match First String(2:w255, 3:w260) -> (0:w256:i32)  [unwired: 1 out]
                n164 = property on="Test Ring" class="Ring (strict)"("Value"=w256, "Strings []"=w255) -> ()  [unwired: 2 in, 2 out]
                n165 = property on="Test Ring" class="Ring (strict)"("Visible"=TRUE) -> ()  [unwired: 2 in, 2 out]
                n166 = property on="Test Slider" class="Slide (strict)"("Visible"=FALSE) -> ()  [unwired: 2 in, 2 out]
              }
              frame "Color Enable  **" {
                n167 = Index Array(array=w267, index=4) -> (element=w268:cluster{string[]})
                n168 = call <vilib>:"NT Read String.vi"("Name"=w270) -> ("String"=w269:string)  [unwired: 9 in, 1 out]
                n169 = Unbundle(w268) -> (w264:string[])
                n170 = Match First String(2:w264, 3:w269) -> (0:w265:i32)  [unwired: 1 out]
                n171 = property on="Test Ring" class="Ring (strict)"("Value"=w265, "Strings []"=w264) -> ()  [unwired: 2 in, 2 out]
                n172 = property on="Test Ring" class="Ring (strict)"("Visible"=TRUE) -> ()  [unwired: 2 in, 2 out]
                n173 = property on="Test Slider" class="Slide (strict)"("Visible"=FALSE) -> ()  [unwired: 2 in, 2 out]
              }
              frame Default {
                n174 = property on="Test Ring" class="Ring (strict)"("Visible"=FALSE) -> ()  [unwired: 2 in, 2 out]
                n175 = property on="Test Slider" class="Slide (strict)"("Visible"=FALSE) -> ()  [unwired: 2 in, 2 out]
              }
              frame "Brightness  **", "Color Level  **", "Compression  **", "FPS  **", "Sharpness  **" {
                n176 = call <vilib>:"NT Read Number.vi"("Name"=w276) -> ("Numeric"=w275:dbl)  [unwired: 9 in, 1 out]
                n177 = local write "Test Slider"(w275) -> ()
                n178 = property on="Test Slider" class="Slide (strict)"("Visible"=TRUE, "Scale.Maximum"=100.0 ("Scale.Range:Maximum")) -> ()  [unwired: 2 in, 2 out]
                n179 = property on="Test Ring" class="Ring (strict)"("Visible"=FALSE) -> ()  [unwired: 2 in, 2 out]
              }
            }
          }
        }
        n180 = property on="Progress" class="Clust (strict)"("Visible"=FALSE) -> ()  [unwired: 2 in, 2 out]
      }
      event "Test Name": Mouse Enter {
        # "Populate the ring with the list of tests"
        n181 = event-data() -> ()  [unwired: 1 in, 1 out]
        n182 = call <vilib>:"NT Read String Array.vi"("Name"="TestMode/TestList") -> ("String Array"=w284:string[])  [unwired: 9 in, 1 out]
        n183 = Build Array (concatenate)("Select the test to run...", w284) -> (w283:string[])
        n184 = property on="Test Name" class="Ring (strict)"("Strings []"=w283) -> ()  [unwired: 2 in, 2 out]
      }
      event "Test Name": Value Change {
        w286 = FALSE ("Visible")
        # "Tell the robot the test name to run"
        n185 = event-data() -> ("NewVal"=w290:u16)  [unwired: 1 in]
        n186 = property on="Test Name" class="Ring (strict)"() -> ("Strings []"=w291:string[])  [unwired: 2 in, 2 out]
        n187 = local write "Progress"(T7 {"Test Progress"=0, "Test Progress Text"=""} ("Progress")) -> ()
        n188 = Index Array(array=w291, index=w290) -> (element=w289:string)
        n189 = call <vilib>:"NT Write String.vi"("String"=w289, "Name"="TestMode/TestName") -> ()  [unwired: 9 in, 1 out]
        n190 = property on="Progress" class="Clust (strict)"("Visible"=TRUE) -> ()  [unwired: 2 in, 2 out]
        n191 = property on="Motor" class="Clust (strict)"("Visible"=w286) -> ()  [unwired: 2 in, 2 out]
        n192 = property on="Test Slider" class="Slide (strict)"("Visible"=w286) -> ()  [unwired: 2 in, 2 out]
        n193 = property on="On/Off" class="Bool (strict)"("Visible"=w286) -> ()  [unwired: 2 in, 2 out]
        n194 = property on="Rev/Fwd" class="Clust (strict)"("Visible"=w286) -> ()  [unwired: 2 in, 2 out]
        n195 = property on="Test Ring" class="Ring (strict)"("Visible"=w286) -> ()  [unwired: 2 in, 2 out]
      }
      event "Listbox": Double Click {
        # "Shift clears all"
        # "Update symbols on the listbox"
        n196 = event-data() -> ("PlatMods.Shift"=w294:bool, "Row"=w296:i32)  [unwired: 1 in]
        n197 = case shown="True" w294 {
          tunnel: w296 -> [w300 _]
          tunnel: 1 -> [w299 _]
          frame False {
            n198 = property on="Listbox" class="LstBox (strict)"() -> ("Item Symbols"=w298:i32[])  [unwired: 2 in, 2 out]
            n199 = Replace Array Subset(array=w298, new element=w299, index=w300) -> (w297:i32[])
            n200 = property on="Listbox" class="LstBox (strict)"("Item Symbols"=w297) -> ()  [unwired: 2 in, 2 out]
          }
          frame True {
            w301 = 0 ("Top Row")
            n201 = property on="Listbox" class="LstBox (strict)"() -> ("Number of Rows"=w303:u32)  [unwired: 2 in, 2 out]
            n202 = Initialize Array(0, w303) -> (w302:i32[])
            n203 = property on="Listbox" class="LstBox (strict)"("Top Row"=w301, "Value"=w301, "Item Symbols"=w302) -> ()  [unwired: 2 in, 2 out]
          }
        }
      }
      event "Listbox": Key Down {
        # "Update symbols on the listbox\nLeft and right keys check and uncheck"
        n204 = event-data() -> ("VKey"=w307:T20)  [unwired: 1 in]
        n205 = case shown="\"Left\", \"Right\"" w307 {
          selector: w307 -> [w312 _]
          tunnel: eventvkey."Left" ("VKey") -> [w310 _]
          frame "Left", "Right" {
            n206 = Equal?(x=w310, y=w312) -> (x = y?=w311:bool)
            n207 = Select(t=0, s=w311, f=1) -> (s? t:f=w313:i32)
            n208 = property on="Listbox" class="LstBox (strict)"() -> ("Item Symbols"=w316:i32[])  [unwired: 2 in, 2 out]
            n209 = Replace Array Subset(array=w316, new element=w313, index="Listbox") -> (w315:i32[])
            n210 = property on="Listbox" class="LstBox (strict)"("Item Symbols"=w315) -> ()  [unwired: 2 in, 2 out]
          }
          frame Default {
          }
        }
      }
      event "DB Camera Config": Value Change {
        # "Show or hide the cluster of controls, store in ini file"
        n211 = event-data() -> ("NewVal"=w320:bool)  [unwired: 1 in]
        n212 = case shown="False" w320 {
          tunnel: w319 -> [w329 _]
          tunnel: [w322 w340] -> w318
          tunnel: w317 -> [w321 w340]
          frame False {
            w336 = "Camera"
            w339 = FALSE ("Visible")
            n213 = local read "Camera Settings"() -> (w328:T2)
            n214 = Index Array(array=w329) -> (element=w332:cluster{string[]})  [unwired: 1 in]
            n215 = Unbundle(w328) -> ("Frame Rate"=w327:i32, "Compression"=w326:i32, "Size"=w330:u16)
            n216 = Unbundle(w332) -> (w331:string[])
            n217 = Index Array(array=w331, index=w330) -> (element=w325:string)
            n218 = call-poly <vilib>:"Write Key.vi"("section"=w336, "value"=w325, "key"="Size", "refnum"=w321) -> ("refnum out"=w338:T18)  [unwired: 2 in, 5 out]
            n219 = call-poly <vilib>:"Write Key.vi"("section"=w336, "value"=w327, "key"="FrameRate", "refnum"=w338) -> ("refnum out"=w337:T18)  [unwired: 1 in, 6 out]
            n220 = property on="Camera Settings" class="Clust (strict)"("Visible"=w339) -> ()  [unwired: 2 in, 2 out]
            n221 = local write "DB Camera Config"(w339) -> ()
            n222 = call-poly <vilib>:"Write Key.vi"("section"=w336, "value"=w326, "key"="Compression", "refnum"=w337) -> ("refnum out"=w323:T18)  [unwired: 1 in, 6 out]
            n223 = call <vilib>:"Close Config Data.vi"("refnum"=w323) -> ("file path"=w324:path)  [unwired: 2 in, 8 out]
            n224 = call <vilib>:"Open Config Data.vi"("configuration file path"=w324) -> ("refnum"=w322:T18)  [unwired: 8 in, 2 out]
          }
          frame True {
            n225 = property on="Camera Settings" class="Clust (strict)"("Visible"=TRUE) -> ()  [unwired: 2 in, 2 out]
          }
        }
      }
      event "Camera Settings": Value Change {
        # "Update summary string when any elements of DB camera change"
        n226 = event-data() -> ("NewVal"=w353:T2)  [unwired: 1 in]
        n227 = Index Array(array=w349) -> (element=w348:cluster{string[]})  [unwired: 1 in]
        n228 = Unbundle(w353) -> ("Frame Rate"=w344:i32, "Compression"=w343:i32, "Size"=w346:u16)
        n229 = Unbundle(w348) -> (w347:string[])
        n230 = Index Array(array=w347, index=w346) -> (element=w345:string)
        n231 = Format Into String(format string="%s   %dfps   %d%%", w345, w344, w343) -> (resulting string=w350:string)  [unwired: 2 in, 1 out]
        n232 = Build Array(w350) -> (w351:string[])
        n233 = property on="DB Camera Config" class="Bool (strict)"("Strings [4]"=w351) -> ()  [unwired: 2 in, 2 out]
      }
      event "Motor.Enable": Value Change {
        # "When the test mode otor enable helper is set, update that\ntree row item's value"
        n234 = event-data() -> ("NewVal"=w359:bool)  [unwired: 1 in]
        n235 = Unbundle("Motor") -> ("Value"=w358:dbl)  [unwired: 1 out]
        n236 = Select(t=w358, s=w359, f=0.0) -> (s? t:f=w356:dbl)
        n237 = call <vilib>:"NT Write Number.vi"("Numeric"=w356, "Name"=w355) -> ()  [unwired: 9 in, 1 out]
      }
      event "Test Slider": Value Change {
        # "When the test mode slider helper is set, update that\ntree row item's value"
        n238 = event-data() -> ("NewVal"=w362:dbl)  [unwired: 1 in]
        n239 = call <vilib>:"NT Write Number.vi"("Numeric"=w362, "Name"=w363) -> ()  [unwired: 9 in, 1 out]
      }
      event "On/Off": Value Change {
        # "When the test mode on/off helper value is set, update that\ntree row item's value"
        n240 = event-data() -> ("NewVal"=w367:bool)  [unwired: 1 in]
        n241 = Boolean To (0,1)(Boolean=w367) -> (0, 1=w366:i16)
        n242 = call <vilib>:"NT Write Number.vi"("Numeric"=w366, "Name"=w365) -> ()  [unwired: 9 in, 1 out]
      }
      event "Rev/Fwd": Value Change {
        # "When the test mode helper value for relays is set, update that\ntree row item's value"
        n243 = event-data() -> ("NewVal.Forward"=w375:bool, "NewVal.Reverse"=w374:bool)  [unwired: 1 in]
        n244 = Boolean To (0,1)(Boolean=w375) -> (0, 1=w371:i16)
        n245 = Boolean To (0,1)(Boolean=w374) -> (0, 1=w373:i16)
        n246 = Negate(x=w373) -> (-x=w372:i16)
        n247 = Add(x=w371, y=w372) -> (x+y=w370:i16)
        n248 = call <vilib>:"NT Write Number.vi"("Numeric"=w370, "Name"=w369) -> ()  [unwired: 9 in, 1 out]
      }
      event "Test Ring": Value Change {
        # "When a test mode helper value is selected from the ring,\nset the tree item's variable to the string value"
        n249 = event-data() -> ("NewVal"=w379:u16)  [unwired: 1 in]
        n250 = property on="Test Ring" class="Ring (strict)"() -> ("Strings []"=w380:string[])  [unwired: 2 in, 2 out]
        n251 = Index Array(array=w380, index=w379) -> (element=w378:string)
        n252 = call <vilib>:"NT Write String.vi"("String"=w378, "Name"=w377) -> ()  [unwired: 9 in, 1 out]
      }
      event "Rec Mode": Value Change {
        # "Update globals for recording mode and path to read log from.\nClear when logging and let NetworkTables set path for vision to\nuse."
        n253 = event-data() -> ("NewVal"=w390:enum32{"Stop", "Record", "Playback"})  [unwired: 1 in]
        n254 = global write "WPI_DashboardLogging Global.vi" "Logging Filename"(path "") -> ()
        n255 = case shown="\"Playback\"" w390 {
          tunnel: w389 -> [_ w392 w400]
          tunnel: [_ _ w399] -> w386
          tunnel: [_ _ w398] -> _
          tunnel: w384 -> [_ _ w396]
          tunnel: cluster{i32, i32} {-250, 170} -> [_ _ w395]
          tunnel: [_ _ T21 {"Image Size"=TRUE, "Image Type"=TRUE, "Pixel Value"=TRUE, "ROI Information"=TRUE, "Zoom Factor"=FALSE} ("Image Information Shown:All Elements")] -> w382
          tunnel: [_ _ TRUE ("Zoom Factor")] -> w381
          frame Default {
          }
          frame "Stop", "Record" {
            # "Place Window too"
            n256 = invoke class="VI" method="FP.Close"(reference=w392) -> (reference out=w391:refnum<vi>)  [unwired: 2 in, 2 out]
            n257 = invoke class="VI" method="Abort VI"(reference=w391) -> ()  [unwired: 2 in, 3 out]
          }
          frame "Playback" {
            n258 = call "Open Playback Panel.vi"("Offset"=w395, "DB VI Ref"=w396, "Playback in"=w400) -> ("Playback out"=w397:refnum<vi>)  [unwired: 8 in]
            n259 = register-events(w397) -> (reference out=w399:refnum<event-registration>, error out=w398:errorcluster)  [unwired: 2 in]
          }
        }
        n260 = global write "WPI_DashboardLogging Global.vi" "Recording"(w390) -> ()
        n261 = property on="Camera Image" class="ImageControl"("Image Information Shown"=w382, "Image Information Visible"=w381) -> ()  [unwired: 2 in, 2 out]
        n262 = call <vilib>:"WPI_DashboardNT Log FieldName Cache.vi"("Operation"=enum16{"Lookup/Add", "Index", "Clear"}."Clear") -> ()  [unwired: 8 in, 3 out]
      }
      event Panel Close {
        w401 = enum32{"Stop", "Record", "Playback"}."Stop" ("Rec Mode")
        # "Playback window has been closed, abort"
        n263 = event-data() -> ()  [unwired: 1 in, 4 out]
        n264 = local write "Rec Mode"(w401) -> ()
        n265 = global write "WPI_DashboardLogging Global.vi" "Recording"(w401) -> ()
      }
      event Panel Close {
        # "Abort playback window and ourself"
        n266 = event-data() -> ()  [unwired: 1 in, 4 out]
        n267 = invoke class="VI" method="FP.Close"(reference=w406) -> (reference out=w405:refnum<vi>)  [unwired: 2 in, 2 out]
        n268 = invoke class="VI" method="Abort VI"(reference=w405) -> (error out=w404:errorcluster)  [unwired: 2 in, 2 out]
        n269 = invoke class="VI" method="Abort VI"(error in=w404) -> ()  [unwired: 2 in, 3 out]
      }
      event "Vision": Value Change {
        # "Enable/Disable Compression slider.\nHW USB is hard-coded into the camera"
        n270 = event-data() -> ("NewVal"=w412:u16)  [unwired: 1 in]
        n271 = Equal?(x=w412, y=u32 2 ("milliseconds to wait")) -> (x = y?=w410:bool)
        n272 = Select(t=T22."Disabled and Grayed Out" ("Disabled"), s=w410, f=T22."Enabled" ("Disabled")) -> (s? t:f=w407:T22)
        n273 = property on="Compression" class="Slide (strict)"("DisabledEnum"=w407) -> ()  [unwired: 2 in, 2 out]
      }
    }
  }
  n274 = while {
    tunnel: w38 -> [w415]
    i -> [w418]
    stop <- FALSE stop-if-true
    n275 = Wait (ms)(milliseconds to wait=u32 100) -> ()  [unwired: 1 out]
    n276 = case shown="\"Playback\"" "Rec Mode" {
      tunnel: w418 -> [_ _ w433]
      tunnel: [u32 2829099 ("Base Color") u32 11141120 ("Target Color") w422] -> w414
      frame "Stop", Default {
        # "Reset the color, extra updates don't cost much"
      }
      frame "Record" {
      }
      frame "Playback" {
        # "Playback"
        n277 = Quotient & Remainder(x=w433, y=u32 50 ("milliseconds to wait")) -> (x-y*floor(x/y)=w429:u32)  [unwired: 1 out]
        n278 = Divide(x=w429, y=u32 50 ("milliseconds to wait")) -> (x/y=w426:dbl)
        n279 = Multiply(x=6.283185307179586, y=w426) -> (x*y=w431:dbl)
        n280 = Sine(x=w431) -> (sin(x)=w430:dbl)
        n281 = Absolute Value(x=w430) -> (abs(x)=w423:dbl)
        n282 = call "Interpolate RGB Color.vi"("Proportion"=w423, "Target Color"=u32 30976, "Base Color"=u32 2829099) -> ("Result Color"=w422:u32)  [unwired: 8 in]
      }
    }
    n283 = property class="Pane"(reference=w415, "PaneColor"=w414) -> ()  [unwired: 1 in, 2 out]
  }
  n284 = TCP Create Listener(10:u16 1741 ("timeout ms (25000)")) -> (3:w1:refnum<k5>)  [unwired: 4 in, 2 out]
  n285 = while {
    tunnel: w1 -> [w435]
    stop <- FALSE stop-if-true
    n286 = TCP Wait On Listener(11:w435) -> (4:w434:refnum<k5>)  [unwired: 3 in, 4 out]
    n287 = local write "TCP"(w434) -> ()
  }
  n288 = property on="On/Off" class="Bool (strict)"("Visible"=w6) -> ()  [unwired: 2 in, 2 out]
  n289 = property on="Motor" class="Clust (strict)"("Visible"=w6) -> ()  [unwired: 2 in, 2 out]
  n290 = property on="Progress" class="Clust (strict)"("Visible"=w6) -> ()  [unwired: 2 in, 2 out]
  n291 = property on="Test Ring" class="Ring (strict)"("Visible"=w6) -> ()  [unwired: 2 in, 2 out]
  n292 = property on="Rev/Fwd" class="Clust (strict)"("Visible"=w6) -> ()  [unwired: 2 in, 2 out]
  n293 = property on="Camera Settings" class="Clust (strict)"("Visible"=w6) -> ()  [unwired: 2 in, 2 out]
  n294 = local write "DB Camera Config"(w6) -> ()
  n295 = global write "WPI_DashboardLogging Global.vi" "Recording"(w32) -> ()
  n296 = local write "Rec Mode"(w32) -> ()
